vi "Collapse Holo On Flatness SLM.vi"(2 "Action":u16(ring) items=["Read", "Initialize"], 5 "collapsed patterns 2":dbl[][](array[numeric]), 7 "collapsed patterns":dbl[][](array[numeric]), 9 "flatness":dbl[][](array[numeric]), 12 "gradient":dbl[][](array[numeric]), 13 "holo mask":dbl[][](array[numeric])) -> (8 "displayed matrix":u8[][](array[numeric]))   [LabVIEW 2014]
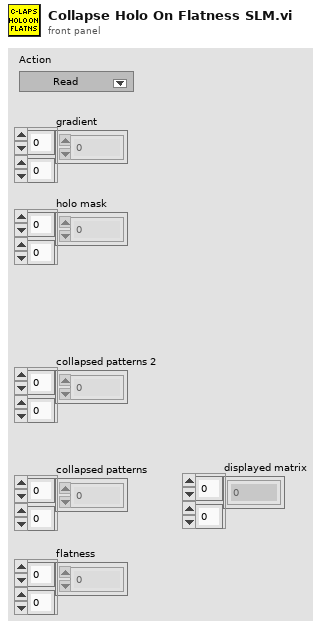
[diagram p1: front panel]
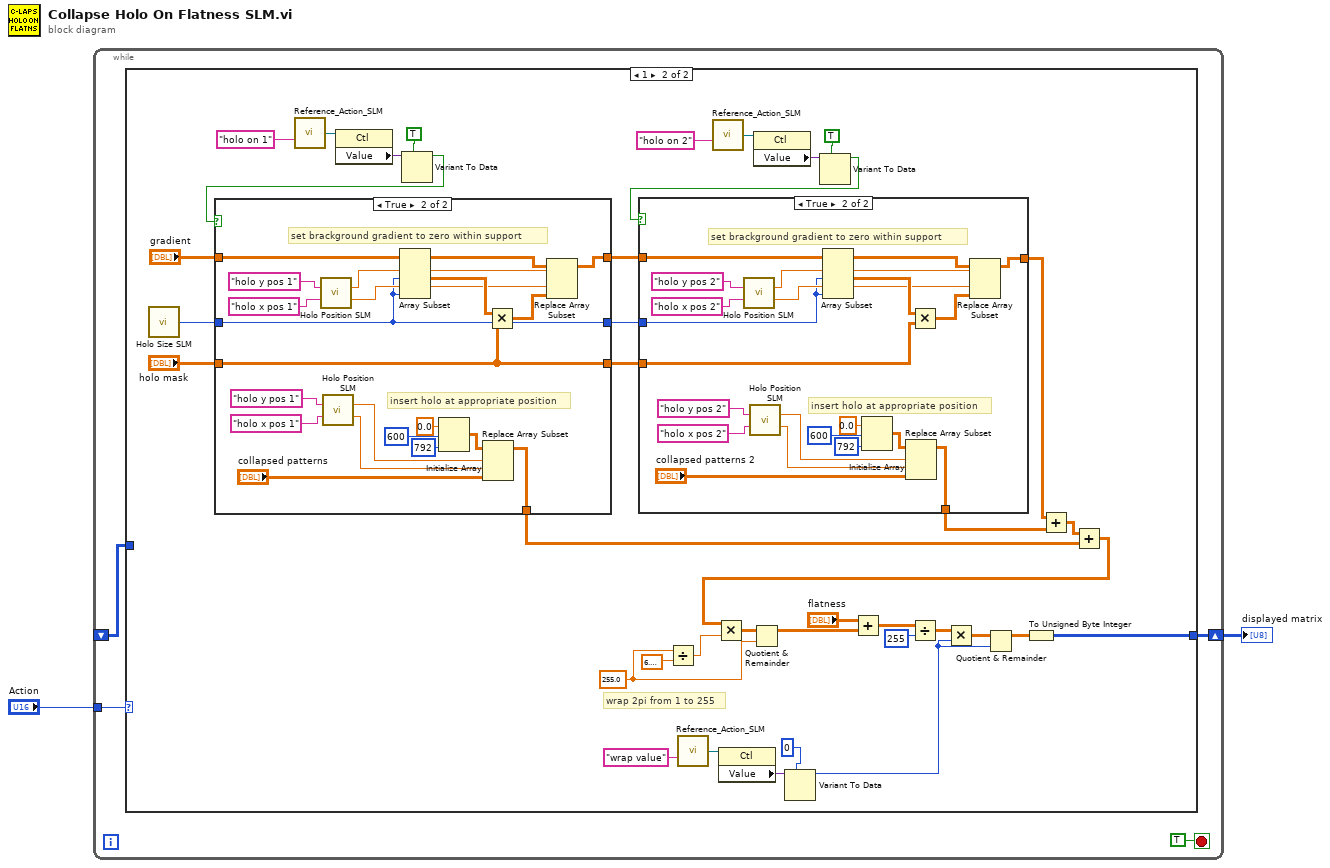
[diagram p0: block diagram]
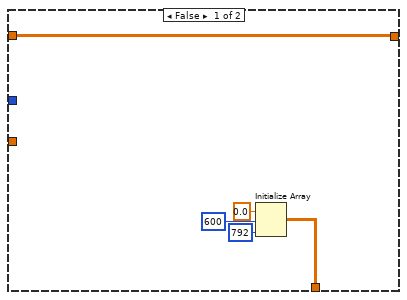
[diagram p3: hidden frame]
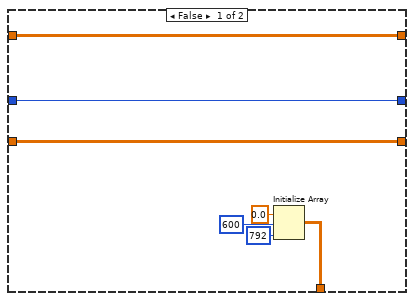
[diagram p4: hidden frame]
diagram:
  n1 = while {
    tunnel: "Action" -> [w5]
    shift-right: [w4] -> w1
    shift-left: _ -> [w3]
    stop <- TRUE stop-if-true
    n2 = case shown="1" w5 {
      tunnel: [w7 w38] -> w4
      tunnel: w3 -> [w7 _]
      frame 0, Default {
      }
      frame 1 {
        w28 = 255.0 ("y")
        # "wrap 2pi from 1 to 255"
        n3 = call "Holo Size SLM.vi"() -> ("data"=w32:i32)  [unwired: 15 in]
        n4 = call "Reference_Action_SLM.vi"("Control Name"="holo on 1") -> ("Ref OUT"=w24:refnum<vi>)  [unwired: 12 in, 2 out]
        n5 = property class="Ctl"(reference=w24) -> ("Value"=w23:variant)  [unwired: 1 in, 2 out]
        n6 = Variant To Data(type=TRUE, Variant=w23) -> (data=w21:bool)  [unwired: 1 in, 1 out]
        n7 = case shown="True" w21 {
          tunnel: "gradient" -> [w77 w94]
          tunnel: [w77 w90] -> w33
          tunnel: w32 -> [w76 w89]
          tunnel: "holo mask" -> [w75 w88]
          tunnel: [w76 w89] -> w20
          tunnel: [w75 w88] -> w19
          tunnel: [w71 w78] -> w12
          frame False {
            n8 = Initialize Array(0.0 ("element"), 600 ("Holo size 2"), 792 ("Holo size 2")) -> (w71:dbl[][])
          }
          frame True {
            # "set brackground gradient to zero within support"
            # "insert holo at appropriate position"
            n9 = call "Holo Position SLM.vi"("y"="holo y pos 1" ("Control Name"), "x"="holo x pos 1" ("Control Name")) -> ("x-y"=w93:dbl, "x-y 2"=w92:dbl)  [unwired: 12 in]
            n10 = call "Holo Position SLM.vi"("y"="holo y pos 1" ("Control Name"), "x"="holo x pos 1" ("Control Name")) -> ("x-y"=w84:dbl, "x-y 2"=w83:dbl)  [unwired: 12 in]
            n11 = Array Subset(array=w94, index (row)=w93, length (row)=w89, index (col)=w92, length (col)=w89) -> (w95:dbl[][])
            n12 = Initialize Array(0.0 ("element"), 600 ("Holo size 2"), 792 ("Holo size 2")) -> (w81:dbl[][])
            n13 = Replace Array Subset(array=w81, new element="collapsed patterns", index (row)=w84, index (col)=w83) -> (w78:dbl[][])
            n14 = Multiply(x=w95, y=w88) -> (x*y=w91:dbl[][])
            n15 = Replace Array Subset(array=w94, new element=w91, index (row)=w93, index (col)=w92) -> (w90:dbl[][])
          }
        }
        n16 = Divide(x=w28, y=6.283185307179586) -> (x/y=w27:dbl)
        n17 = call "Reference_Action_SLM.vi"("Control Name"="wrap value") -> ("Ref OUT"=w42:refnum<vi>)  [unwired: 12 in, 2 out]
        n18 = call "Reference_Action_SLM.vi"("Control Name"="holo on 2") -> ("Ref OUT"=w18:refnum<vi>)  [unwired: 12 in, 2 out]
        n19 = property class="Ctl"(reference=w42) -> ("Value"=w41:variant)  [unwired: 1 in, 2 out]
        n20 = property class="Ctl"(reference=w18) -> ("Value"=w17:variant)  [unwired: 1 in, 2 out]
        n21 = Variant To Data(type=0, Variant=w41) -> (data=w40:i32)  [unwired: 1 in, 1 out]
        n22 = Variant To Data(type=TRUE, Variant=w17) -> (data=w15:bool)  [unwired: 1 in, 1 out]
        n23 = case shown="True" w15 {
          tunnel: w33 -> [w50 w66]
          tunnel: [w50 w63] -> w14
          tunnel: w20 -> [_ w62]
          tunnel: w19 -> [_ w61]
          tunnel: [w46 w51] -> w13
          frame False {
            n24 = Initialize Array(0.0 ("element"), 600 ("Holo size 2"), 792 ("Holo size 2")) -> (w46:dbl[][])
          }
          frame True {
            # "set brackground gradient to zero within support"
            # "insert holo at appropriate position"
            n25 = call "Holo Position SLM.vi"("y"="holo y pos 2" ("Control Name"), "x"="holo x pos 2" ("Control Name")) -> ("x-y"=w69:dbl, "x-y 2"=w68:dbl)  [unwired: 12 in]
            n26 = call "Holo Position SLM.vi"("y"="holo y pos 2" ("Control Name"), "x"="holo x pos 2" ("Control Name")) -> ("x-y"=w59:dbl, "x-y 2"=w58:dbl)  [unwired: 12 in]
            n27 = Array Subset(array=w66, index (row)=w69, length (row)=w62, index (col)=w68, length (col)=w62) -> (w70:dbl[][])
            n28 = Initialize Array(0.0 ("element"), 600 ("Holo size 2"), 792 ("Holo size 2")) -> (w54:dbl[][])
            n29 = Replace Array Subset(array=w54, new element="collapsed patterns 2", index (row)=w59, index (col)=w58) -> (w51:dbl[][])
            n30 = Multiply(x=w70, y=w61) -> (x*y=w67:dbl[][])
            n31 = Replace Array Subset(array=w66, new element=w67, index (row)=w69, index (col)=w68) -> (w63:dbl[][])
          }
        }
        n32 = Add(x=w14, y=w13) -> (x+y=w11:dbl[][])
        n33 = Add(x=w11, y=w12) -> (x+y=w10:dbl[][])
        n34 = Multiply(x=w10, y=w27) -> (x*y=w26:dbl[][])
        n35 = Quotient & Remainder(x=w26, y=w28) -> (x-y*floor(x/y)=w25:dbl[][])  [unwired: 1 out]
        n36 = Add(x="flatness", y=w25) -> (x+y=w39:dbl[][])
        n37 = Divide(x=w39, y=u8 255) -> (x/y=w44:dbl[][])
        n38 = Multiply(x=w44, y=w40) -> (x*y=w36:dbl[][])
        n39 = Quotient & Remainder(x=w36, y=w40) -> (x-y*floor(x/y)=w35:dbl[][])  [unwired: 1 out]
        n40 = To Unsigned Byte Integer(number=w35) -> (unsigned 8bit integer=w38:u8[][])
      }
    }
  }
  "displayed matrix" <- w1
